vi "RT-Mode-Selection.vi"(1 "Array":dbl[](array[numeric])) -> (0 "Numeric":u64)   [LabVIEW 2020]
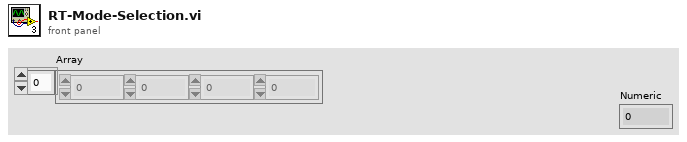
[diagram p1: front panel]
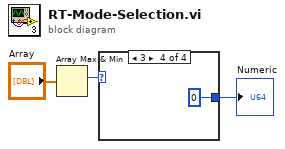
[diagram p0: block diagram]
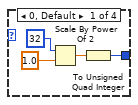
[diagram p2: hidden frame]
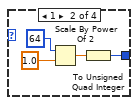
[diagram p3: hidden frame]
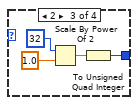
[diagram p4: hidden frame]
diagram:
  n1 = Array Max & Min(array="Array") -> (max index (indices)=w2:i32)  [unwired: 3 out]
  n2 = case shown="3" w2 {
    tunnel: [w5 w9 w12 u64 0] -> w1
    frame 0, Default {
      n3 = Scale By Power Of 2(n=i16 32, x=1.0) -> (x*2^n=w4:dbl)
      n4 = To Unsigned Quad Integer(1:w4) -> (0:w5:u64)
    }
    frame 1 {
      n5 = Scale By Power Of 2(n=i16 64, x=1.0) -> (x*2^n=w8:dbl)
      n6 = To Unsigned Quad Integer(1:w8) -> (0:w9:u64)
    }
    frame 2 {
      n7 = Scale By Power Of 2(n=i16 32, x=1.0) -> (x*2^n=w13:dbl)
      n8 = To Unsigned Quad Integer(1:w13) -> (0:w12:u64)
    }
    frame 3 {
    }
  }
  "Numeric" <- w1
